vi "Make dPWM JSON.vi"(9 "Force":bool, 10 "Tmpl values":T1={"type"="AI", "device"="", "name"="", "data"={"<init"=FALSE, "<duty_cycle"=0.0, "<dio_pin"=0.0}}, 11 "Tmpl values":T1={"type"="AI", "device"="", "name"="", "data"={"<init"=FALSE, "<duty_cycle"=0.0, "<dio_pin"=0.0}}) -> (3 "delta JSON":string)   [LabVIEW 2019]
uses:
  dPWM Data proto.ctl
  dPWM proto.ctl
panel:
  out "Complete JSON":string
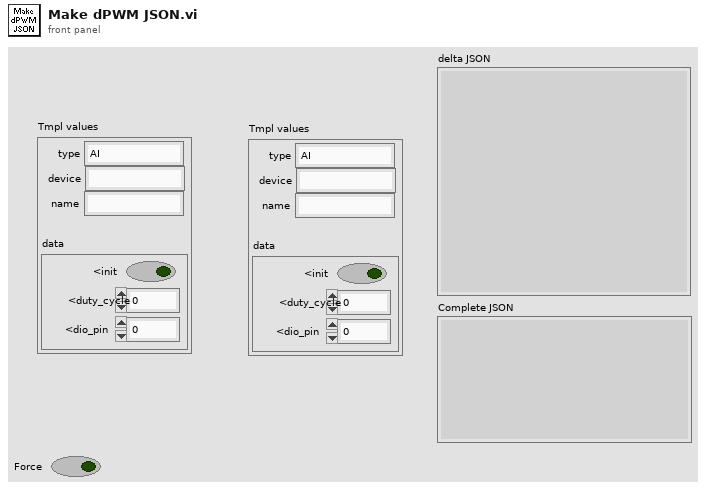
[diagram p1: front panel]
types:
  T1 = typedef "dPWM proto.ctl" = cluster{"type":string, "device":string, "name":string, "data":T2}
  T2 = typedef "dPWM Data proto.ctl" = cluster{"<init":bool, "<duty_cycle":dbl, "<dio_pin":dbl}
  T3 = cluster{"type":bool, "device":bool, "name":bool, "data":cluster{"<init":bool, "<duty_cycle":bool, "<dio_pin":bool}}
  T4 = cluster{"<init":bool, "<duty_cycle":bool, "<dio_pin":bool}
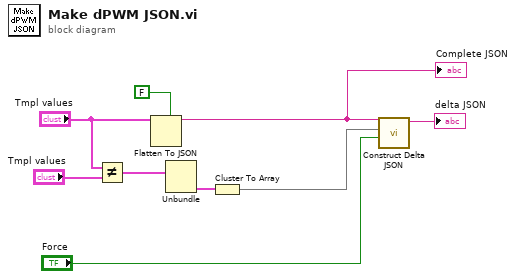
[diagram p0: block diagram]
diagram:
  n1 = Not Equal?(x="Tmpl values", y="Tmpl values") -> (x != y?=w6:T3)
  n2 = Flatten To JSON(enable LabVIEW extensions? (T)=FALSE, anything="Tmpl values") -> (JSON string=w5:string)  [unwired: 1 in, 1 out]
  "Complete JSON" <- w5
  n3 = Unbundle(w6) -> ("data"=w2:T4)  [unwired: 3 out]
  n4 = Cluster To Array(cluster=w2) -> (array=w1:bool[])
  n5 = call "Construct Delta JSON.vi"("Force"="Force", "Checked Items"=w1, "JSON string"=w5) -> ("Delta JSON"=→"delta JSON":string)  [unwired: 8 in]
